vi "Contact Report (SubVI).vi"(0 "reportPath_ref":refnum<vi>, 1 "SampleIDref":refnum<vi>, 2 "Shot Graph":refnum<vi>) -> ()   [LabVIEW 2012]
uses:
  <vilib>/Utility/NIReport.llb/NI_report.lvclass
  <vilib>/Utility/NIReport.llb/Append Report Text (str wrap).vi
  <vilib>/Utility/NIReport.llb/Append Text Table to Report (wrap).vi
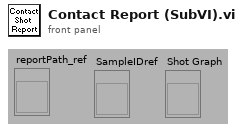
[diagram p1: front panel]
types:
  T1 = enum16{"Standard Report", "HTML", "Word", "Excel"}
  T2 = cluster{"Charset (-1)":i16, "Weight (-1)":i16, "Name":string, "Size":string}
  T3 = cluster{"Italic":enum16{"Italic Unchanged", "Italic On", "Italic Off"}, "Strike Through":enum16{"Strike Through Unchanged", "Strike Through On", "Strike Through Off"}, "Underline":enum16{"Underline Unchanged", "Underline On", "Underline Off"}, "Bold":enum16{"Bold Unchanged", "Bold On", "Bold Off"}}
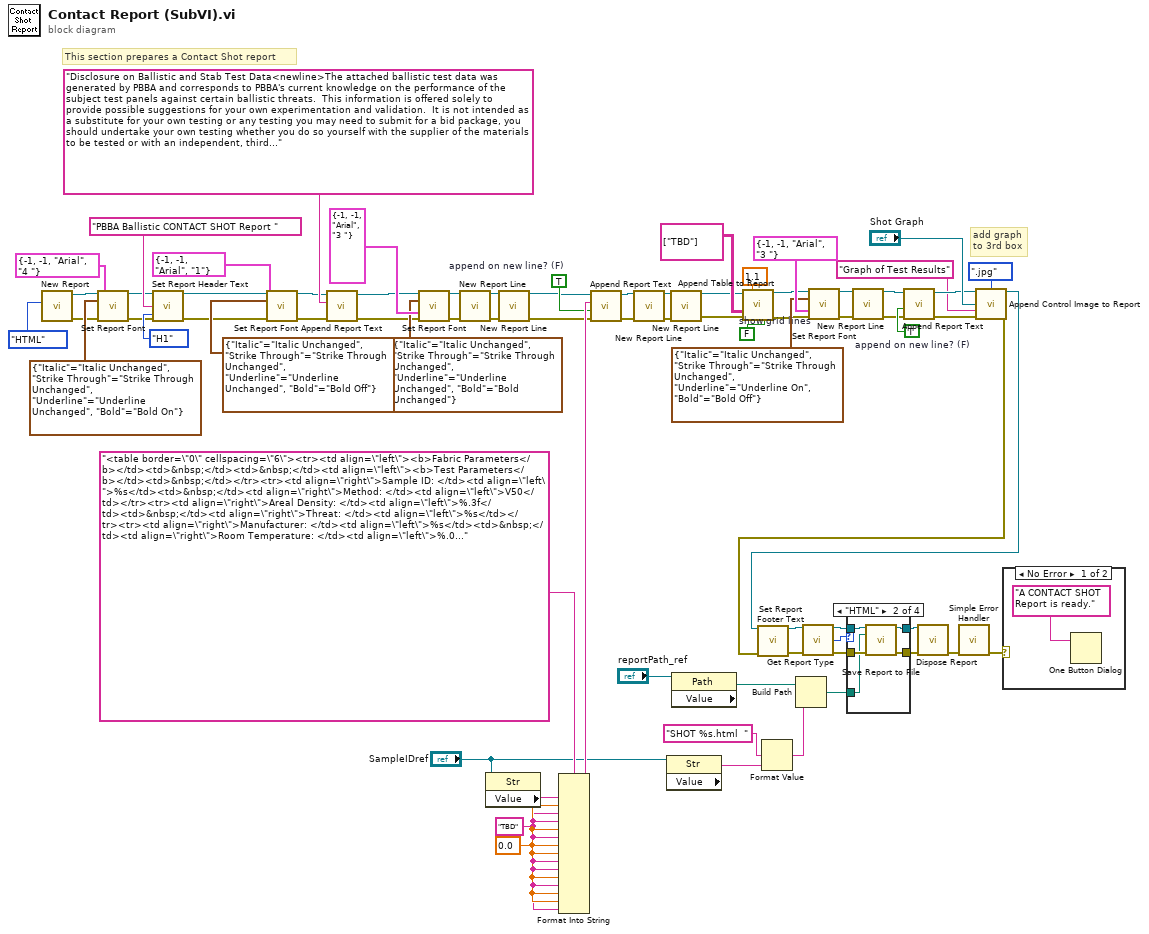
[diagram p0: block diagram]
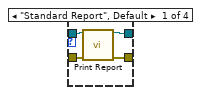
[diagram p3: hidden frame]
diagram:
  w59 = "TBD" ("Input 2")
  w69 = 0.0 ("Input 1")
  w49 = TRUE  # append on new line? (F)
  w36 = TRUE  # append on new line? (F)
  w12 = FALSE  # show grid lines
  # "This section prepares a Contact Shot report"
  # "add graph to 3rd box"
  n1 = call <vilib>:"New Report.vi"("report type"=T1."HTML") -> ("report out"=w10:refnum<class "NI_report.lvclass">, "error out"=w11:errorcluster)  [unwired: 13 in]
  n2 = call-dynamic "Set Report Font.vi"("report in"=w10, "text options"=T3 {"Italic"=enum."Italic Unchanged", "Strike Through"=enum."Strike Through Unchanged", "Underline"=enum."Underline Unchanged", "Bold"=enum."Bold On"}, "font settings"=T2 {"Charset (-1)"=-1, "Weight (-1)"=-1, "Name"="Arial", "Size"="4 "}, "error in (no error)"=w11) -> ("report out"=w26:refnum<class "NI_report.lvclass">, "error out"=w25:errorcluster)  [unwired: 9 in, 1 out]
  n3 = call-dynamic "Set Report Header Text.vi"("report in"=w26, "center header text"="PBBA Ballistic CONTACT SHOT Report ", "error in (no error)"=w25, "HTML header size"=enum16{"H1", "H2", "H3", "H4", "H5", "H6", "H7"}."H1") -> ("report out"=w23:refnum<class "NI_report.lvclass">, "error out"=w22:errorcluster)  [unwired: 10 in]
  n4 = call-dynamic "Set Report Font.vi"("report in"=w23, "text options"=T3 {"Italic"=enum."Italic Unchanged", "Strike Through"=enum."Strike Through Unchanged", "Underline"=enum."Underline Unchanged", "Bold"=enum."Bold Off"}, "font settings"=T2 {"Charset (-1)"=-1, "Weight (-1)"=-1, "Name"="Arial", "Size"="1"}, "error in (no error)"=w22) -> ("report out"=w38:refnum<class "NI_report.lvclass">, "error out"=w37:errorcluster)  [unwired: 9 in, 1 out]
  n5 = call-poly <vilib>:"Append Report Text.vi"("report in"=w38, "text"="Disclosure on Ballistic and Stab Test Data<newline>The attached ballistic test data was generated by PBBA and corresponds to PBBA's current knowledge on the performance of the subject test panels against certain ballistic threats.  This information is offered solely to provide possible suggestions for your own experimentation and validation.  It is not intended as a substitute for your own testing or any testing you may need to submit for a bid package, you should undertake your own testing whether you do so yourself with the supplier of the materials to be tested or with an independent, third party, certified testing facility and the supplier of the materials to be tested (i.e., the fabric weaver).  PBBA makes no warranties, and assumes no liabilities in connection with any use of the information supplied with this disclosure statement.", "error in (no error)"=w37) -> ("report out"=w39:refnum<class "NI_report.lvclass">, "error out"=w41:errorcluster)  [unwired: 9 in, 2 out]
  n6 = call-dynamic "Set Report Font.vi"("report in"=w39, "text options"=T3 {"Italic"=enum."Italic Unchanged", "Strike Through"=enum."Strike Through Unchanged", "Underline"=enum."Underline Unchanged", "Bold"=enum."Bold Unchanged"}, "font settings"=T2 {"Charset (-1)"=-1, "Weight (-1)"=-1, "Name"="Arial", "Size"="3 "}, "error in (no error)"=w41) -> ("report out"=w40:refnum<class "NI_report.lvclass">, "error out"=w42:errorcluster)  [unwired: 9 in, 1 out]
  n7 = call-dynamic "New Report Line.vi"("report in"=w40, "error in (no error)"=w42) -> ("report out"=w9:refnum<class "NI_report.lvclass">, "error out"=w8:errorcluster)  [unwired: 12 in]
  n8 = property class="Str"(reference="SampleIDref") -> ("Value"=w70:string)  [unwired: 1 in, 2 out]
  n9 = call-dynamic "New Report Line.vi"("report in"=w9, "error in (no error)"=w8) -> ("report out"=w34:refnum<class "NI_report.lvclass">, "error out"=w35:errorcluster)  [unwired: 12 in]
  n10 = Format Into String(format string="<table border=\"0\" cellspacing=\"6\"><tr><td align=\"left\"><b>Fabric Parameters</b></td><td>&nbsp;</td><td>&nbsp;</td><td align=\"left\"><b>Test Parameters</b></td><td>&nbsp;</td></tr><tr><td align=\"right\">Sample ID: </td><td align=\"left\">%s</td><td>&nbsp;</td><td align=\"right\">Method: </td><td align=\"left\">V50</td></tr><tr><td align=\"right\">Areal Density: </td><td align=\"left\">%.3f</td><td>&nbsp;</td><td align=\"right\">Threat: </td><td align=\"left\">%s</td></tr><tr><td align=\"right\">Manufacturer: </td><td align=\"left\">%s</td><td>&nbsp;</td><td align=\"right\">Room Temperature: </td><td align=\"left\">%.0f</td></tr><tr><td align=\"right\">Group Data: </td><td align=\"left\">%s</td><td>&nbsp;</td><td align=\"right\">Correction Factor: </td><td align=\"left\">%0.4f</td></tr><tr><td align=\"right\">Projectile Weight: </td><td align=\"left\">%0.3f</td><td>&nbsp;</td><td align=\"right\">Panel Backing: </td><td align=\"left\">%s</td></tr><tr><td align=\"right\">Powder Type: </td><td align=\"left\">%s</td><td>&nbsp;</td><td align=\"right\">Shot Angle: </td><td align=\"left\">%.0f</td></tr><tr><td align=\"right\">Test Conditions: </td><td align=\"left\">%s</td><td>&nbsp;</td><td align=\"right\">Room Humidity: </td><td align=\"left\">%.0f</td></tr><tr><td align=\"right\">Panel Weight: </td><td align=\"left\">%.4f</td><td>&nbsp;</td><td>&nbsp;</td></tr><tr><td align=\"right\">Descripton: </td><td align=\"left\">%s</td><td>&nbsp;</td><td>&nbsp;</td></tr></table>", w70, w69, w59, w59, w69, w59, w69, w69, w59, w59, w69, w59, w69, w69, w59) -> (resulting string=w50:string)  [unwired: 2 in, 1 out]
  n11 = call-poly <vilib>:"Append Report Text.vi"("report in"=w34, "text"=w50, "append on new line? (F)"=w36, "error in (no error)"=w35) -> ("report out"=w55:refnum<class "NI_report.lvclass">, "error out"=w54:errorcluster)  [unwired: 8 in, 2 out]
  n12 = call-dynamic "New Report Line.vi"("report in"=w55, "error in (no error)"=w54) -> ("report out"=w15:refnum<class "NI_report.lvclass">, "error out"=w14:errorcluster)  [unwired: 12 in]
  n13 = property class="Str"(reference="SampleIDref") -> ("Value"=w68:string)  [unwired: 1 in, 2 out]
  n14 = call-dynamic "New Report Line.vi"("report in"=w15, "error in (no error)"=w14) -> ("report out"=w16:refnum<class "NI_report.lvclass">, "error out"=w17:errorcluster)  [unwired: 12 in]
  n15 = property class="Path"(reference="reportPath_ref") -> ("Value"=w67:path)  [unwired: 1 in, 2 out]
  n16 = call-poly <vilib>:"Append Table to Report.vi"("report in"=w16, "column width (1)"=1.1, "text data"=string[][] [["TBD"]], "error in (no error)"=w17, "show grid lines"=w12) -> ("report out"=w48:refnum<class "NI_report.lvclass">, "error out"=w44:errorcluster)  [unwired: 7 in, 2 out]
  n17 = Format Value(format string="SHOT %s.html  " ("string (\"\")"), value (0)=w68) -> (output string=w31:string)  [unwired: 1 in]
  n18 = Build Path(base path=w67, name or relative path=w31) -> (appended path=w33:path)
  n19 = call-dynamic "Set Report Font.vi"("report in"=w48, "text options"=T3 {"Italic"=enum."Italic Unchanged", "Strike Through"=enum."Strike Through Unchanged", "Underline"=enum."Underline On", "Bold"=enum."Bold Off"}, "font settings"=T2 {"Charset (-1)"=-1, "Weight (-1)"=-1, "Name"="Arial", "Size"="3 "}, "error in (no error)"=w44) -> ("report out"=w47:refnum<class "NI_report.lvclass">, "error out"=w46:errorcluster)  [unwired: 9 in, 1 out]
  n20 = call-dynamic "New Report Line.vi"("report in"=w47, "error in (no error)"=w46) -> ("report out"=w18:refnum<class "NI_report.lvclass">, "error out"=w19:errorcluster)  [unwired: 12 in]
  n21 = call-poly <vilib>:"Append Report Text.vi"("report in"=w18, "append on new line? (F)"=w49, "error in (no error)"=w19) -> ("report out"=w57:refnum<class "NI_report.lvclass">, "error out"=w58:errorcluster)  [unwired: 9 in, 2 out]
  n22 = call-dynamic "Append Control Image to Report.vi"("report in"=w57, "image file type (.jpg)"=enum16{".jpg", ".png"}.".jpg" ("image file type(.png)"), "ctrl reference"="Shot Graph", "description"="Graph of Test Results" ("control name"), "error in (no error)"=w58) -> ("report out"=w72:refnum<class "NI_report.lvclass">, "error out"=w71:errorcluster)  [unwired: 7 in, 2 out]
  n23 = call-dynamic "Set Report Footer Text.vi"("report in"=w72, "error in (no error)"=w71) -> ("report out"=w21:refnum<class "NI_report.lvclass">, "error out"=w20:errorcluster)  [unwired: 12 in]
  n24 = call-dynamic "Get Report Type.vi"("report in"=w21, "error in (no error)"=w20) -> ("report out"=w6:refnum<class "NI_report.lvclass">, "report type"=w7:T1, "error out"=w3:errorcluster)  [unwired: 11 in]
  n25 = case shown="\"HTML\"" w7 {
    tunnel: w6 -> [w77 w82 w83 w86]
    tunnel: [w76 w81 w83 w86] -> w5
    tunnel: [w75 w80 w84 w85] -> w4
    tunnel: w3 -> [w74 w79 w84 w85]
    tunnel: w33 -> [_ w78 _ _]
    frame "Standard Report", Default {
      n26 = call-dynamic "Print Report.vi"("report in"=w77, "error in (no error)"=w74) -> ("report out"=w76:refnum<class "NI_report.lvclass">, "error out"=w75:errorcluster)  [unwired: 12 in]
    }
    frame "HTML" {
      n27 = call-dynamic "Save Report to File.vi"("report in"=w82, "report file path"=w78, "error in (no error)"=w79) -> ("report out"=w81:refnum<class "NI_report.lvclass">, "error out"=w80:errorcluster)  [unwired: 11 in]
    }
    frame "Word" {
    }
    frame "Excel" {
    }
  }
  n28 = call-dynamic "Dispose Report.vi"("report in"=w5, "error in (no error)"=w4) -> ("error out"=w53:errorcluster)  [unwired: 13 in]
  n29 = call <vilib>:"Simple Error Handler.vi"("error in (no error)"=w53) -> ("error out"=w52:errorcluster)  [unwired: 4 in, 4 out]
  n30 = case shown="No Error" w52 {
    frame No Error {
      n31 = One Button Dialog(message="A CONTACT SHOT Report is ready.") -> ()  [unwired: 1 in, 1 out]
    }
    frame Error {
    }
  }
